vi "RegionGrow.vi"(4 "gray Image":T1(plugin-control), 5 "Color Image":T1(plugin-control)) -> (1 "Image grow":T1(plugin-control), 2 "颜色（2g-r-b）":i32)   [LabVIEW 2015]
uses:
  Realse/Nebogrow.dll
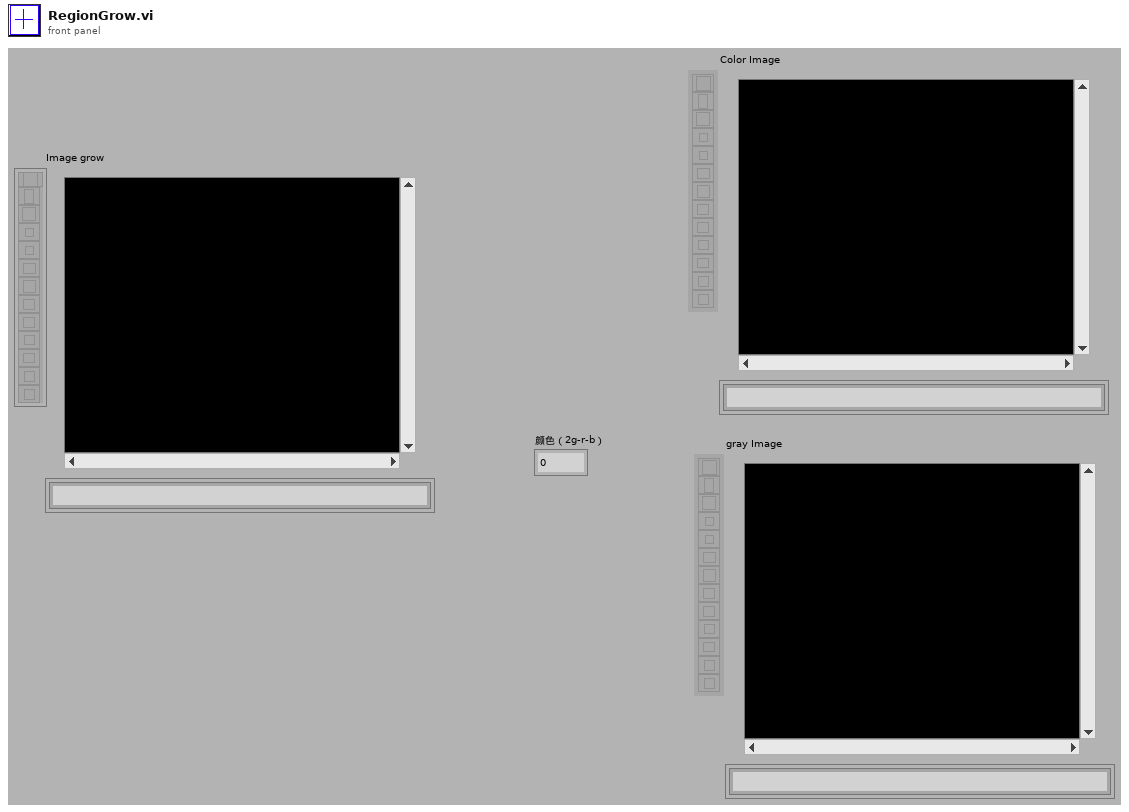
[diagram p1: front panel]
types:
  T1 = typedef "IMAQ Image.ctl" = refnum<image>
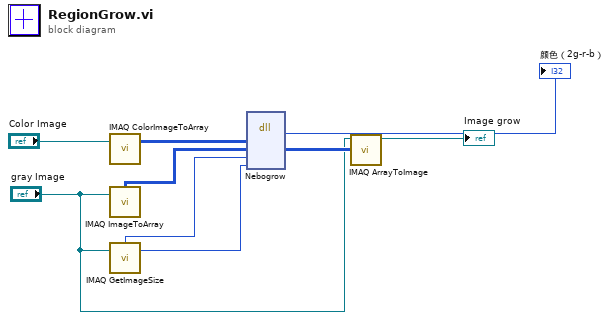
[diagram p0: block diagram]
diagram:
  n1 = call "IMAQ ColorImageToArray"("Image"="Color Image") -> ("Image Pixels (U32)"=w9:u32[][])  [unwired: 2 in, 3 out]
  n2 = call "IMAQ ImageToArray"("Image"="gray Image") -> ("Image Pixels (U8)"=w5:u8[][])  [unwired: 2 in, 5 out]
  n3 = call "IMAQ GetImageSize"("Image"="gray Image") -> ("Y Resolution"=w6:i32, "X Resolution"=w7:i32)  [unwired: 1 in, 3 out]
  n4 = dll-call lib="PTH2eabs E文章投稿&51. 代明球老师-玉米胁迫实验\tRGB程序maizeRealseNebogrow.dll" fn="Nebogrow"("pImag"=w9, "Graybuff"=w5, "width"=w7, "height"=w6) -> ("return type"=→"颜色（2g-r-b）":i32, "Graybuff"=w4:u8[][])  [unwired: 6 in, 2 out]
  n5 = call "IMAQ ArrayToImage"("Image Pixels (U8)"=w4, "Image"="gray Image") -> ("Image Out"=→"Image grow":T1)  [unwired: 4 in, 5 out]
